vi "Set g.vi"(10 "g":dbl, 11 "AbstractDstarNode in":refnum<class "NI_Robotics_AbstractDstarNode.lvclass">) -> (3 "AbstractDstarNode out":refnum<class "NI_Robotics_AbstractDstarNode.lvclass">)   [LabVIEW 2017, in "NI_Robotics_AbstractDstarNode.lvclass"]
uses:
  <vilib>/robotics/Navigation/shared/MapNode/AbstractDstarNode/NI_Robotics_AbstractDstarNode.lvclass
  <vilib>/robotics/Navigation/shared/MapNode/AbstractDstarNode/NI_Robotics_AbstractDstarNode.lvclass/NI_Robotics_AbstractDstarNode.ctl
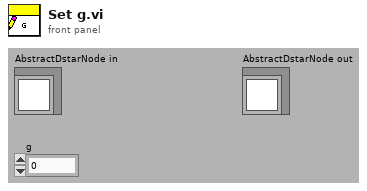
[diagram p1: front panel]
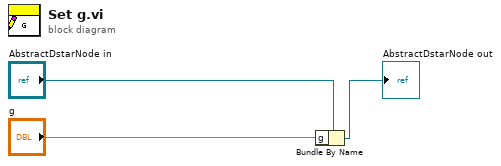
[diagram p0: block diagram]
diagram:
  n1 = Bundle By Name(cluster="AbstractDstarNode in", "g"="g") -> (→"AbstractDstarNode out":refnum<class "NI_Robotics_AbstractDstarNode.lvclass">)
